vi "Main.vi"(11 "Module Admin":refnum<class "Delacor_lib_QMH_Module Admin.lvclass">) -> ()   [LabVIEW 2019, in "ACQ.lvlib"]
doc: "This template is based off of the Queued Message Handler design pattern and the Queued Message Handler project template that ships with LabVIEW.\n\nThe main difference is that the queue is private to this module and communication between modules is performed via Broadcast and Request events.\n\nRequest events are wrapped in public API methods and are handled in the Event Handling Loop (EHL) of this VI. Any module can register for Broadcast events sent by this module. The EHL generates messages based on user interface actions.\n\nThe Message Handling Loop (MHL) processes messages generated by the EHL, or by other messages. The messages are string values, so new messages can be added easily to the Message Cases case structure in the MHL. Each message cluster can also provide an optional value for Message Data, which is a variant that can be converted to whatever message-specific data is required.\n_____\nBased on Delacor QMH Project Template 5.0.0.82."
uses:
  ACQ.lvlib
  <vilib>/Delacor/Delacor QMH/Libraries/Module Admin_class/Delacor_lib_QMH_Module Admin.lvclass
  Module Data--cluster.ctl
  stop helper loop Argument--cluster.ctl
  <vilib>/Delacor/Delacor QMH/Libraries/Message Queue_class/Delacor_lib_QMH_Message Queue.lvclass/Delacor_lib_QMH_Message Queue.ctl
  Stop Argument--cluster.ctl
  <vilib>/Delacor/Delacor QMH/Libraries/Module Admin_class/Delacor_lib_QMH_Module Admin.lvclass/Delacor_lib_QMH_Module Admin.ctl
  start acquiere Argument--cluster.ctl
  stop acquiere Argument--cluster.ctl
  <vilib>/Utility/miscctls.llb/LVPointTypeDef.ctl
  <vilib>/Delacor/Delacor QMH/Libraries/Message Queue_class/Delacor_lib_QMH_Enqueue Message (Single).vi
  <vilib>/Delacor/Delacor QMH/Libraries/Module Admin_class/Delacor_lib_QMH_Get External Launch.vi
  <vilib>/Utility/error.llb/Error Cluster From Error Code.vi
  <vilib>/ErrorRing/Error Ring.xnode
  <vilib>/Delacor/Delacor QMH/Libraries/Message Queue_class/Delacor_lib_QMH_Message Queue.lvclass
panel:
  out "Waveform Graph":dynamicdata(graph)
  out "Time Stamp":timestamp
  in  "Simulate MHL Error":bool
  in  "Simulate EHL Error":bool
  out "error out":errorcluster
  out "Status":string
  # "Other QMH Modules communicate with this Module via its Public API (wrappers for its Request Events).\n\nThis Module communicates with other Modules via its Broadcast Events.\nAny module that wants to get these messages, just registers for this module's Broadcast events."
  # "This template is for the Delacor Modified Queued Message Handler design pattern.\n\nSee the block diagram for more information on how to use this template."
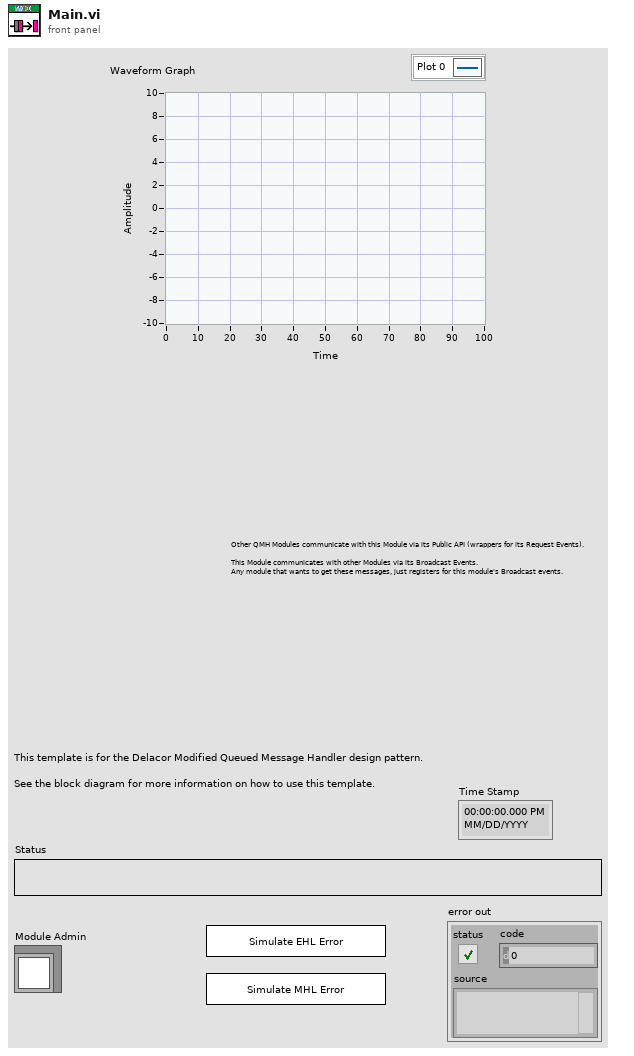
[diagram p1: front panel]
types:
  T1 = typedef "ACQ.lvlib/Request Events--cluster.ctl" = cluster{"Stop Module":refnum<user-event>, "Show Panel":refnum<user-event>, "Hide Panel":refnum<user-event>, "Get Module Execution Status":refnum<user-event>, "Show Diagram":refnum<user-event>, "Start helper loop":refnum<user-event>, "stop helper loop":refnum<user-event>, "start acquiere":refnum<user-event>, "stop acquiere":refnum<user-event>}
  T2 = typedef "ACQ.lvlib/Module Data--cluster.ctl" = cluster{"Status":string}
  T3 = typedef "ACQ.lvlib/stop helper loop Argument--cluster.ctl" = cluster{"Boolean":bool}
  T4 = enum32{"invalid lock state", "Not Locked", "Locked (No Password)", "Password-protected"}
  T5 = typedef "ACQ.lvlib/start acquiere Argument--cluster.ctl" = cluster{"Boolean":bool}
  T6 = typedef "ACQ.lvlib/stop acquiere Argument--cluster.ctl" = cluster{"Boolean":bool}
  T7 = typedef "LVPointTypeDef.ctl" = cluster{"Horizontal":i16, "Vertical":i16}
  T8 = enum32{"Invalid", "Standard", "Closed", "Hidden", "Minimized", "Maximized"}
  T9 = typedef "ACQ.lvlib/Stop Argument--cluster.ctl" = cluster{"Origin":string, "Exit via Stop Module Req?":bool, "Wait for Module to stop?":bool}
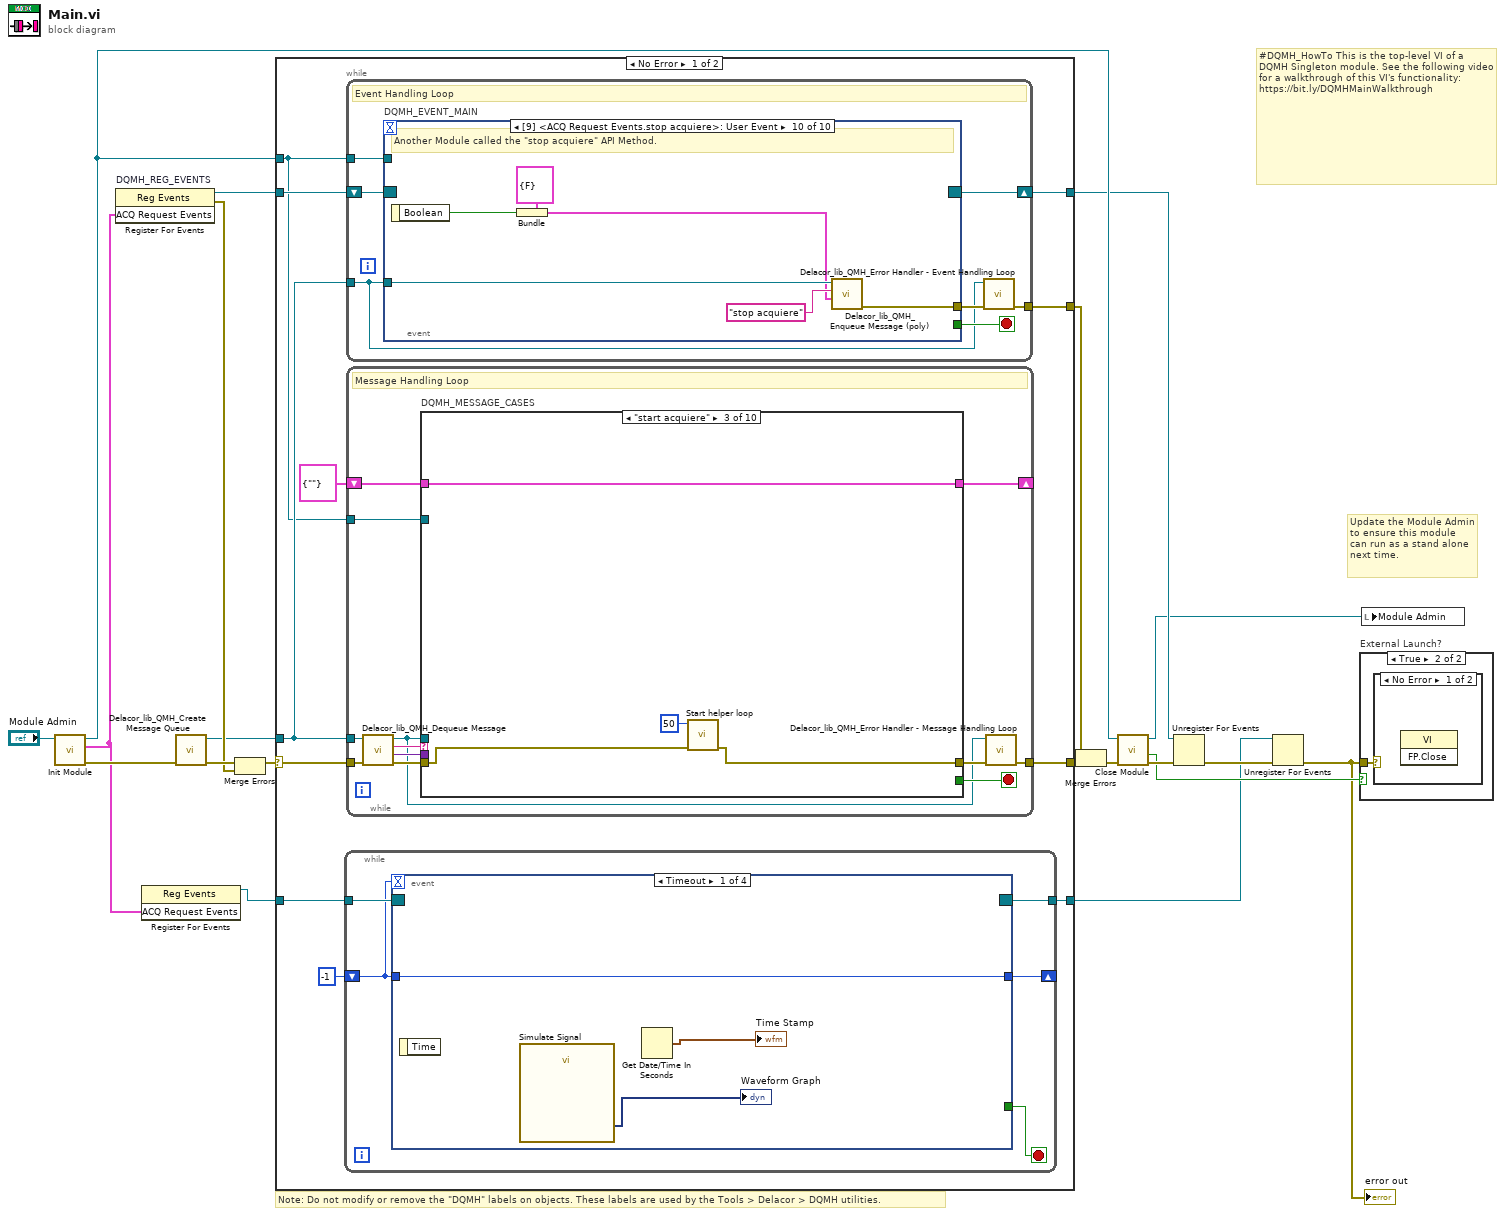
[diagram p0: block diagram]
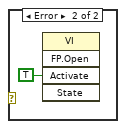
[diagram p3: hidden frame]
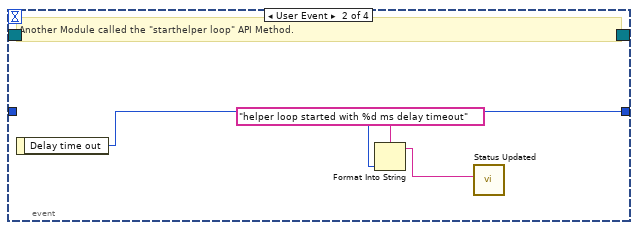
[diagram p4: hidden frame]
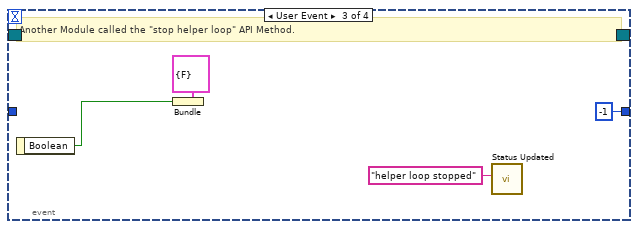
[diagram p5: hidden frame]
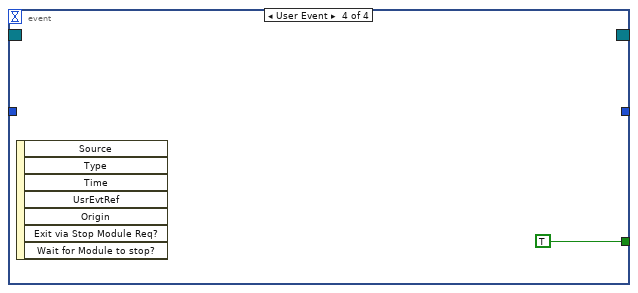
[diagram p6: hidden frame]
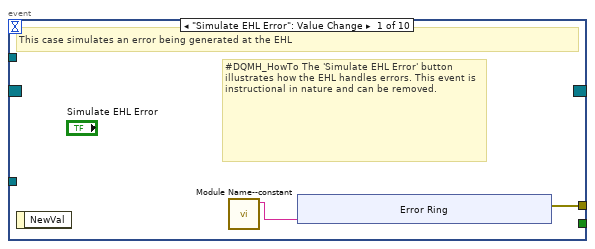
[diagram p7: hidden frame]
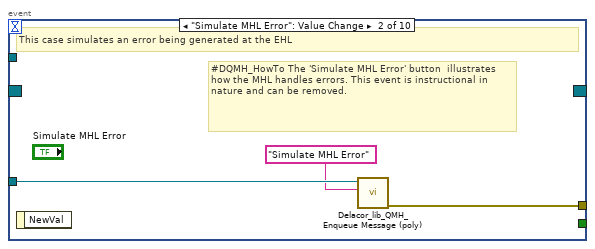
[diagram p8: hidden frame]
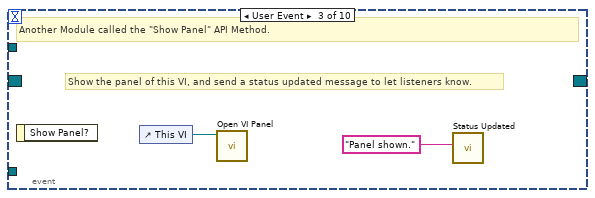
[diagram p9: hidden frame]
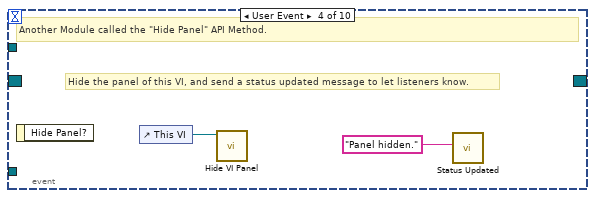
[diagram p10: hidden frame]
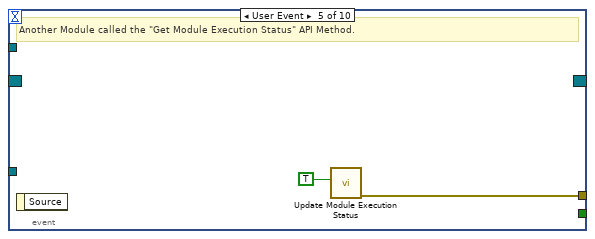
[diagram p11: hidden frame]
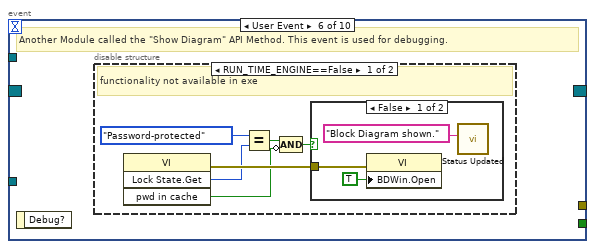
[diagram p12: hidden frame]
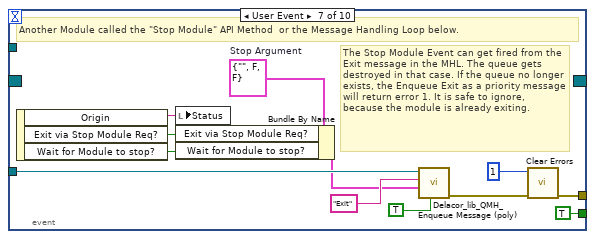
[diagram p15: hidden frame]
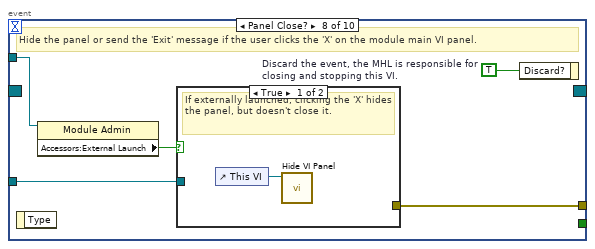
[diagram p16: hidden frame]
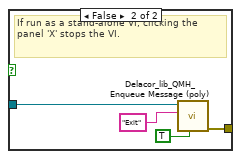
[diagram p17: hidden frame]
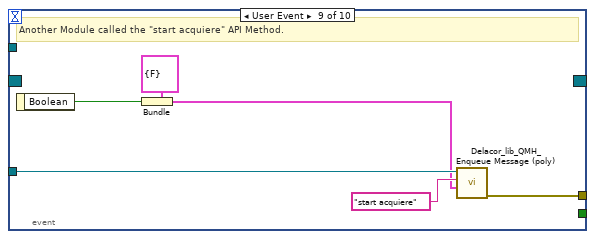
[diagram p18: hidden frame]
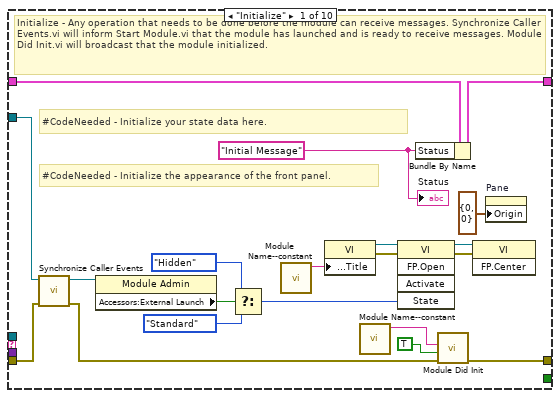
[diagram p19: hidden frame]
diagram:
  # "#DQMH_HowTo This is the top-level VI of a DQMH Singleton module. See the following video for a walkthrough of this VI's functionality: https://bit.ly/DQMHMainWalkthrough"
  # "Note: Do not modify or remove the \"DQMH\" labels on objects. These labels are used by the Tools > Delacor > DQMH utilities."
  # "Update the Module Admin to ensure this module can run as a stand alone next time."
  n1 = call "Init Module.vi"("Singleton Module Admin in"="Module Admin") -> ("error out"=w19:errorcluster, "ACQ Request Events"=w4:T1, "Singleton Module Admin out"=w12:refnum<class "Delacor_lib_QMH_Module Admin.lvclass">)  [unwired: 8 in]
  n2 = register-events "DQMH_REG_EVENTS"(w4) -> (reference out=w10:refnum<event-registration>, error out=w13:errorcluster)  [unwired: 2 in]
  n3 = register-events(w4) -> (reference out=w5:refnum<event-registration>)  [unwired: 2 in, 1 out]
  n4 = call <vilib>:"Delacor_lib_QMH_Create Message Queue.vi"("error in (no error)"=w19) -> ("error out"=w15:errorcluster, "Message Queue"=w9:refnum<class "Delacor_lib_QMH_Message Queue.lvclass">)  [unwired: 9 in]
  n5 = Merge Errors(w15, w13) -> (w14:errorcluster)
  n6 = case shown="No Error" w14 {
    selector: w14 -> [w29 w227]
    tunnel: [w31 w226] -> w20
    tunnel: [w28 w232] -> w11
    tunnel: w10 -> [w26 w232]
    tunnel: w9 -> [w25 w225]
    tunnel: [w30 _] -> w17
    tunnel: w12 -> [w24 w228]
    tunnel: w5 -> [w23 w224]
    tunnel: [w22 w224] -> w1
    frame No Error {
      n7 = while {
        tunnel: w23 -> [w36]
        tunnel: [w35] -> w22
        shift-right: [w33] -> _
        shift-left: -1 -> [w32]
        stop <- w34 stop-if-true
        n8 = event shown="[0] Timeout" {
          selector: w36 -> [_ _ _ _]
          dyn-events: [_ _ _ _] -> w35
          timeout: w32 -> [_ _ _ _]
          tunnel: [_ _ _ TRUE] -> w34
          tunnel: [w39 w42 -1 _] -> w33
          tunnel: w32 -> [w39 _ _ _]
          event Timeout {
            n9 = event-data() -> ()  [unwired: 1 in, 1 out]
            n10 = call "Simulate Signal"() -> ("Sine"=→"Waveform Graph":dynamicdata)  [unwired: 14 in, 1 out]
            n11 = Get Date/Time In Seconds() -> (seconds since 1Jan1904=→"Time Stamp":timestamp)
          }
          event User Event {
            # "Another Module called the \"starthelper loop\" API Method."
            n12 = event-data() -> ("Delay time out"=w42:i32)  [unwired: 1 in]
            n13 = Format Into String(format string="helper loop started with %d ms delay timeout", w42) -> (resulting string=w41:string)  [unwired: 2 in, 1 out]
            n14 = call "Status Updated.vi"("Status"=w41) -> ()  [unwired: 10 in, 1 out]
          }
          event User Event {
            # "Another Module called the \"stop helper loop\" API Method."
            n15 = event-data() -> ("Boolean"=w45:bool)  [unwired: 1 in]
            n16 = Bundle(cluster=T3 {"Boolean"=FALSE} ("stop helper loop Argument"), "Boolean"=w45) -> ()  [unwired: 1 out]
            n17 = call "Status Updated.vi"("Status"="helper loop stopped") -> ()  [unwired: 10 in, 1 out]
          }
          event User Event {
            n18 = event-data() -> ()  [unwired: 1 in, 7 out]
          }
        }
      }
      n19 = while {
        tunnel: w25 -> [w48]
        shift-right: [w51] -> w28
        shift-left: w26 -> [w52]
        tunnel: [w53] -> w30
        tunnel: w24 -> [w49]
        stop <- w50 stop-if-true
        # "Event Handling Loop"
        n20 = event "DQMH_EVENT_MAIN" shown="[9] <ACQ Request Events.stop acquiere>: User Event" {
          selector: w52 -> [_ _ _ _ _ _ _ _ _ _]
          dyn-events: [_ _ _ _ _ _ _ _ _ _] -> w51
          timeout: _ -> [_ _ _ _ _ _ _ _ _ _]
          tunnel: [_ _ _ _ _ _ TRUE ("Discard?") _ _ _] -> w50
          tunnel: w48 -> [_ w65 _ _ _ _ w89 w96 w109 w115]
          tunnel: [w56 w66 _ _ w72 _ w92 w98 w104 w110] -> w54
          tunnel: w49 -> [_ _ _ _ _ _ _ w95 _ _]
          event "Simulate EHL Error": Value Change {
            # "#DQMH_HowTo The 'Simulate EHL Error' button  illustrates how the EHL handles errors. This event is instructional in nature and can be removed."
            # "This case simulates an error being generated at the EHL"
            n21 = event-data() -> ()  [unwired: 1 in, 1 out]
            n22 = call "Module Name--constant.vi"() -> ("Module Name"=w55:string)  [unwired: 11 in]
            n23 = xnode "Error Ring"("parameter 0"=w55) -> ("error out"=w56:errorcluster)
          }
          event "Simulate MHL Error": Value Change {
            # "#DQMH_HowTo The 'Simulate MHL Error' button  illustrates how the MHL handles errors. This event is instructional in nature and can be removed."
            # "This case simulates an error being generated at the EHL"
            n24 = event-data() -> ()  [unwired: 1 in, 1 out]
            n25 = call-poly <vilib>:"Delacor_lib_QMH_Enqueue Message (poly).vi"("Message"="Simulate MHL Error", "Message Queue in"=w65) -> ("error out"=w66:errorcluster)  [unwired: 8 in, 1 out]
          }
          event User Event {
            # "Show the panel of this VI, and send a status updated message to let listeners know."
            # "Another Module called the \"Show Panel\" API Method."
            n26 = event-data() -> ()  [unwired: 1 in, 1 out]
            n27 = control-ref of="This VI"() -> (w68:refnum<vi>)
            n28 = call "Open VI Panel.vi"("VI"=w68) -> ()  [unwired: 10 in, 1 out]
            n29 = call "Status Updated.vi"("Status"="Panel shown." ("format string")) -> ()  [unwired: 10 in, 1 out]
          }
          event User Event {
            # "Hide the panel of this VI, and send a status updated message to let listeners know."
            # "Another Module called the \"Hide Panel\" API Method."
            n30 = event-data() -> ()  [unwired: 1 in, 1 out]
            n31 = control-ref of="This VI"() -> (w70:refnum<vi>)
            n32 = call "Hide VI Panel.vi"("VI"=w70) -> ()  [unwired: 10 in, 1 out]
            n33 = call "Status Updated.vi"("Status"="Panel hidden." ("format string")) -> ()  [unwired: 10 in, 1 out]
          }
          event User Event {
            # "Another Module called the \"Get Module Execution Status\" API Method."
            n34 = event-data() -> ()  [unwired: 1 in, 1 out]
            n35 = call "Update Module Execution Status.vi"("Running?"=TRUE) -> ("error out"=w72:errorcluster)  [unwired: 10 in]
          }
          event User Event {
            # "Another Module called the \"Show Diagram\" API Method. This event is used for debugging."
            n36 = event-data() -> ()  [unwired: 1 in, 1 out]
            n37 = disable-structure shown="RUN_TIME_ENGINE==False" {
              frame condition #0 (active) {
                # "functionality not available in exe"
                n38 = invoke class="VI" method="Lock State.Get"() -> (error out=w78:errorcluster, "Get Lock State"=w77:T4, "pwd in cache"=w74:bool)  [unwired: 4 in, 1 out]
                n39 = Equal?(x=T4."Password-protected", y=w77) -> (x = y?=w75:bool)
                n40 = Compound Arithmetic op=AND(w75, invert w74) -> (w73:bool)
                n41 = case shown="False" w73 {
                  tunnel: w78 -> [w81 _]
                  frame False {
                    n42 = property class="VI"(error in=w81, "BDWin.Open"=TRUE ("Block Diagram Window:Open")) -> ()  [unwired: 1 in, 2 out]
                    n43 = call "Status Updated.vi"("Status"="Block Diagram shown." ("format string")) -> ()  [unwired: 10 in, 1 out]
                  }
                  frame True {
                    # "Password-protected VI, and the password is not in the cache. Do not show the diagram."
                  }
                }
              }
              frame condition #1 {
              }
            }
          }
          event User Event {
            w85 = T9 {"Origin"="", "Exit via Stop Module Req?"=FALSE, "Wait for Module to stop?"=FALSE}  # Stop Argument
            # "The Stop Module Event can get fired from the Exit message in the MHL. The queue gets destroyed in that case. If the queue no longer exists, the Enqueue Exit as a priority message will return error 1. It is safe to ignore, because the module is already exiting."
            # "Another Module called the \"Stop Module\" API Method  or the Message Handling Loop below."
            n44 = event-data() -> ("Origin"=w88:string, "Exit via Stop Module Req?"=w84:bool, "Wait for Module to stop?"=w83:bool)  [unwired: 1 in]
            n45 = local write "Status"(w88) -> ()
            n46 = Bundle By Name(cluster=w85, "Exit via Stop Module Req?"=w84, "Wait for Module to stop?"=w83) -> (w82:T9)
            n47 = call-poly <vilib>:"Delacor_lib_QMH_Enqueue Message (poly).vi"("Priority Message? (F)"=TRUE, "Message Data"=w82, "Message"="Exit", "Message Queue in"=w89) -> ("error out"=w93:errorcluster)  [unwired: 6 in, 1 out]
            n48 = call <vilib>:"Clear Errors.vi"("error in (no error)"=w93, "specific error code to clear (0: all)"=1) -> ("error out"=w92:errorcluster)  [unwired: 4 in, 1 out]
          }
          event Panel Close? {
            w97 = TRUE  # Discard the event, the MHL is responsible for closing and stopping this VI.
            # "Hide the panel or send the 'Exit' message if the user clicks the 'X' on the module main VI panel."
            n49 = event-data() -> ()  [unwired: 1 in, 1 out]
            n50 = property class="Module Admin"(reference=w95) -> ("Accessors:External Launch"=w94:bool)  [unwired: 1 in, 2 out]
            n51 = case shown="True" w94 {
              tunnel: w96 -> [_ w102]
              tunnel: [_ w103] -> w98
              frame True {
                # "If externally launched, clicking the 'X' hides the panel, but doesn't close it."
                n52 = control-ref of="This VI"() -> (w99:refnum<vi>)
                n53 = call "Hide VI Panel.vi"("VI"=w99) -> ()  [unwired: 10 in, 1 out]
              }
              frame False {
                # "If run as a stand-alone VI, clicking the panel 'X' stops the VI."
                n54 = call-poly <vilib>:"Delacor_lib_QMH_Enqueue Message (poly).vi"("Priority Message? (F)"=TRUE, "Message"="Exit", "Message Queue in"=w102) -> ("error out"=w103:errorcluster)  [unwired: 7 in, 1 out]
              }
            }
            n55 = event-data("Discard?"=w97) -> ()  [unwired: 1 in, 1 out]
          }
          event User Event {
            # "Another Module called the \"start acquiere\" API Method."
            n56 = event-data() -> ("Boolean"=w105:bool)  [unwired: 1 in]
            n57 = Bundle(cluster=T5 {"Boolean"=FALSE} ("start acquiere Argument"), "Boolean"=w105) -> (w106:T5)
            n58 = call-poly <vilib>:"Delacor_lib_QMH_Enqueue Message (poly).vi"("Message Data"=w106, "Message"="start acquiere", "Message Queue in"=w109) -> ("error out"=w104:errorcluster)  [unwired: 7 in, 1 out]
          }
          event User Event {
            # "Another Module called the \"stop acquiere\" API Method."
            n59 = event-data() -> ("Boolean"=w111:bool)  [unwired: 1 in]
            n60 = Bundle(cluster=T6 {"Boolean"=FALSE} ("stop acquiere Argument"), "Boolean"=w111) -> (w112:T6)
            n61 = call-poly <vilib>:"Delacor_lib_QMH_Enqueue Message (poly).vi"("Message Data"=w112, "Message"="stop acquiere", "Message Queue in"=w115) -> ("error out"=w110:errorcluster)  [unwired: 7 in, 1 out]
          }
        }
        n62 = call-dynamic "Delacor_lib_QMH_Error Handler - Event Handling Loop.vi"("error in (no error)"=w54, "Message Queue in"=w48) -> ("dup error in"=w53:errorcluster)  [unwired: 8 in, 1 out]
      }
      n63 = while {
        tunnel: w25 -> [w118]
        shift-right: [w122] -> _
        shift-left: T2 {"Status"=""} ("Data Cluster") -> [w123]
        tunnel: w29 -> [w126]
        tunnel: [w124] -> w31
        tunnel: w24 -> [w116]
        stop <- w121 stop-if-true
        # "Message Handling Loop"
        n64 = call-dynamic "Delacor_lib_QMH_Dequeue Message.vi"("error in (no error)"=w126, "Message Queue in"=w118) -> ("error out"=w125:errorcluster, "Message Data"=w119:variant, "Message"=w120:string, "Message Queue out"=w117:refnum<class "Delacor_lib_QMH_Message Queue.lvclass">)  [unwired: 6 in]
        n65 = case "DQMH_MESSAGE_CASES" shown="\"start acquiere\"" w120 {
          selector: w120 -> [_ _ _ _ _ _ _ _ _ w211]
          tunnel: w117 -> [_ _ _ _ _ _ _ w181 w203 _]
          tunnel: w125 -> [w145 w149 w152 w160 w163 w165 w170 w188 w209 w213]
          tunnel: [w143 w149 w151 w154 w162 w165 w169 w184 w206 w214] -> w127
          tunnel: w123 -> [w134 w148 w153 w159 w161 w164 w167 w183 w202 w212]
          tunnel: [w133 w148 w153 w159 w161 w164 w167 w183 w202 w212] -> w122
          tunnel: [_ _ _ _ _ _ _ _ w201 _] -> w121
          tunnel: w119 -> [_ _ _ w158 _ _ _ w182 w200 _]
          tunnel: w116 -> [w135 _ _ _ _ _ _ w180 w195 _]
          frame "Initialize" {
            w128 = "Initial Message" ("Initial Message")
            # "#CodeNeeded - Initialize the appearance of the front panel."
            # "#CodeNeeded - Initialize your state data here."
            # "Initialize - Any operation that needs to be done before the module can receive messages. Synchronize Caller Events.vi will inform Start Module.vi that the module has launched and is ready to receive messages. Module Did Init.vi will broadcast that the module initialized."
            n66 = call "Synchronize Caller Events.vi"("error in (no error)"=w145, "Singleton Module Admin in"=w135) -> ("error out"=w144:errorcluster, "Singleton Module Admin out"=w130:refnum<class "Delacor_lib_QMH_Module Admin.lvclass">)  [unwired: 8 in]
            n67 = property class="Module Admin"(reference=w130) -> ("Accessors:External Launch"=w139:bool)  [unwired: 1 in, 2 out]
            n68 = Select(t=T8."Hidden" ("State"), s=w139, f=T8."Standard" ("State")) -> (s? t:f=w136:T8)
            n69 = call "Module Name--constant.vi"() -> ("Module Name"=w142:string)  [unwired: 11 in]
            n70 = property class="VI"("Front Panel.Title"=w142) -> (reference out=w141:refnum<vi>, error out=w147:errorcluster)  [unwired: 2 in]
            n71 = call "Module Name--constant.vi"() -> ("Module Name"=w131:string)  [unwired: 11 in]
            n72 = invoke class="VI" method="FP.Open"(reference=w141, error in=w147, "State"=w136) -> (reference out=w140:refnum<vi>, error out=w146:errorcluster)  [unwired: 2 in, 3 out]
            n73 = Bundle By Name(cluster=w134, "Status"=w128) -> (w133:T2)
            n74 = call "Module Did Init.vi"("error in (no error)"=w144, "Initialized?"=TRUE, "Origin"=w131) -> ("error out"=w143:errorcluster)  [unwired: 8 in]
            n75 = invoke class="VI" method="FP.Center"(reference=w140, error in=w146) -> ()  [unwired: 1 in, 3 out]
            n76 = property on="Pane" class="Pane"("Origin"=T7 {"Horizontal"=0, "Vertical"=0}) -> ()  [unwired: 2 in, 2 out]
            "Status" <- w128
          }
          frame "--- Module Specific ---" {
            # "Separator -- The following cases handle messages specific to this Module."
          }
          frame "start acquiere" {
            n77 = call "Start helper loop.vi"("error in (no error)"=w152, "Delay time out"=50) -> ("error out"=w151:errorcluster)  [unwired: 9 in]
          }
          frame "stop acquiere" {
            # "#CodeNeeded\n1. Configure this Message Case for handling the \"stop acquiere\" message.\n2. Delete or edit this label when done."
            n78 = Variant To Data(error in=w160, type=T6 {"Boolean"=FALSE} ("stop acquiere Argument"), Variant=w158) -> (data=w156:T6, error out=w155:errorcluster)
            n79 = Unbundle By Name(w156) -> ()  [unwired: 1 out]
            n80 = call "stop acquiere.vi"("error in (no error)"=w155) -> ("error out"=w154:errorcluster)  [unwired: 10 in]
          }
          frame "---Copy This Frame---" {
            # "Duplicate this frame when creating new messages.  Change this comment in the duplicated frame to describe this message."
            n81 = Merge Errors(w163) -> (w162:errorcluster)
          }
          frame "--- Exit and Error Handling---" {
            # "Separator - The following cases handle errors and exit messages."
          }
          frame "Simulate MHL Error" {
            # "#DQMH_HowTo The 'Simulate MHL Error' button  illustrates how the MHL handles errors. This event is instructional in nature and can be removed."
            # "Simulate an error occurring at the MHL"
            n82 = call "Module Name--constant.vi"() -> ("Module Name"=w166:string)  [unwired: 11 in]
            n83 = xnode "Error Ring"("parameter 0"=w166) -> ("error out"=w168:errorcluster)
            n84 = Merge Errors(w170, w168) -> (w169:errorcluster)
          }
          frame "Error" {
            # "#CodeRecommended - If you ever change the name of this \"Error\" message, you'll need to update the name in the Check Loop Error.vi as well."
            # "#CodeRecommended - If the module is running in standalone mode (External Launch = FALSE), this code will pop up an error dialog and call the 'Exit' message if an error occurs. Add more fine-grained error handling here."
            # "Error - Check the error message data and respond accordingly. This message is sent by the \"Error Handler\" VIs at the end of each loop in this application."
            n85 = property class="Module Admin"(reference=w180) -> ("Accessors:External Launch"=w179:bool)  [unwired: 1 in, 2 out]
            n86 = Variant To Data(error in=w188, type=errorcluster {"status"=FALSE, "code"=0, "source"=""} ("error constant"), Variant=w182) -> (data=w189:errorcluster, error out=w186:errorcluster)
            n87 = call "Module Name--constant.vi"() -> ("Module Name"=w178:string)  [unwired: 11 in]
            n88 = call "Error Reported.vi"("Additional Information"=w178, "Error"=w189) -> ()  [unwired: 9 in, 1 out]
            n89 = case shown="False" w179 {
              tunnel: [w194 _] -> w185
              tunnel: w181 -> [w192 _]
              tunnel: w189 -> [w193 _]
              frame False {
                # "If the module is running standalone, then pop up an error dialog and call the \"Exit\" message."
                n90 = call <vilib>:"Simple Error Handler.vi"("error in (no error)"=w193) -> ()  [unwired: 4 in, 5 out]
                n91 = call-poly <vilib>:"Delacor_lib_QMH_Enqueue Message (poly).vi"("Priority Message? (F)"=TRUE, "Message"="Exit", "Message Queue in"=w192) -> ("error out"=w194:errorcluster)  [unwired: 7 in, 1 out]
              }
              frame True {
                # "If the module was launched externally, calling the Error Reported broadcast VI is the only action performed by the \"Error\" message. The module's caller can then process the error appropriately."
              }
            }
            n92 = Merge Errors(w186, w185) -> (w184:errorcluster)
            n93 = local write "error out"(w184) -> ()
          }
          frame "Exit" {
            w199 = 91  # 91: not all Exit messages will have an argument
            w201 = TRUE  # Stop the VI
            # "Release the message queue reference"
            # "#CodeNeeded - Add any required cleanup code here"
            # "Exit - Exit the application."
            n94 = Variant To Data(error in=w209, type=T9 {"Origin"="", "Exit via Stop Module Req?"=FALSE, "Wait for Module to stop?"=FALSE} ("Stop Argument"), Variant=w200) -> (data=w197:T9, error out=w205:errorcluster)
            n95 = call <vilib>:"Clear Errors.vi"("error in (no error)"=w205, "specific error code to clear (0: all)"=w199) -> ("error out"=w208:errorcluster)  [unwired: 4 in, 1 out]
            n96 = control-ref of="This VI"() -> (w196:refnum<vi>)
            n97 = call-dynamic "Delacor_lib_QMH_Release Message Queue.vi"("error in (no error)"=w208, "Message Queue"=w203) -> ("error out"=w207:errorcluster)  [unwired: 9 in]
            n98 = call "Handle Exit.vi"("Stop Argument"=w197, "Admin in"=w195, "VI reference"=w196) -> ("error out"=w204:errorcluster)  [unwired: 7 in, 1 out]
            n99 = Merge Errors(w207, w204) -> (w206:errorcluster)
          }
          frame Default {
            # "'Default' case only runs if there is a message that isn't defined in any of the other cases.  Output a programming error."
            n100 = call "Module Name--constant.vi"() -> ("Module Name"=w210:string)  [unwired: 11 in]
            n101 = xnode "Error Ring"("parameter 0"=w211, "parameter 1"=w210) -> ("error out"=w215:errorcluster)
            n102 = Merge Errors(w213, w215) -> (w214:errorcluster)
          }
        }
        n103 = call-dynamic "Delacor_lib_QMH_Error Handler - Message Handling Loop.vi"("error in (no error)"=w127, "Message Queue in"=w117) -> ("dup error in"=w124:errorcluster)  [unwired: 8 in, 1 out]
      }
    }
    frame Error {
      # "Synchronize Caller Events.vi will inform Start Module.vi that the module has launched and will let the code calling Start Module.vi register for broadcasts and would permit the caller receive the broadcast that an error occurred at launch time."
      n104 = call-dynamic "Delacor_lib_QMH_Release Message Queue.vi"("error in (no error)"=w227, "Message Queue"=w225) -> ("error out"=w226:errorcluster)  [unwired: 9 in]
      n105 = call "Synchronize Caller Events.vi"("Singleton Module Admin in"=w228) -> ("error out"=w233:errorcluster)  [unwired: 9 in, 1 out]
      n106 = call "Module Name--constant.vi"() -> ("Module Name"=w231:string)  [unwired: 11 in]
      n107 = Format Into String(format string="An error occurred during initialization. %s is no longer running.", w231) -> (resulting string=w229:string)  [unwired: 2 in, 1 out]
      n108 = Merge Errors(w226, w233) -> (w234:errorcluster)
      n109 = call "Error Reported.vi"("Additional Information"=w229, "Error"=w234) -> ()  [unwired: 9 in, 1 out]
    }
  }
  n110 = Merge Errors(w17, w20) -> (w16:errorcluster)
  n111 = call "Close Module.vi"("error in (no error)"=w16, "Module Admin in"=w12) -> ("error out"=w18:errorcluster, "External Launch"=w6:bool, "Module Admin out"=w7:refnum<class "Delacor_lib_QMH_Module Admin.lvclass">)  [unwired: 7 in]
  n112 = Unregister For Events(event registration refnum=w11, error in=w18) -> (error out=w3:errorcluster)
  n113 = Unregister For Events(event registration refnum=w1, error in=w3) -> (error out=w2:errorcluster)
  "error out" <- w2
  n114 = case "External Launch?" shown="True" w6 {
    tunnel: w2 -> [_ w235]
    frame False {
    }
    frame True {
      n115 = case shown="No Error" w235 {
        frame No Error {
          n116 = invoke class="VI" method="FP.Close"() -> ()  [unwired: 3 in, 3 out]
        }
        frame Error {
          n117 = invoke class="VI" method="FP.Open"("Activate"=TRUE ("Activate?")) -> ()  [unwired: 4 in, 5 out]
        }
      }
    }
  }
  n118 = local write "Module Admin"(w7) -> ()
